vi "Set all current limits (SubVI).vi"() -> (3 "String":string)   [LabVIEW 2018]
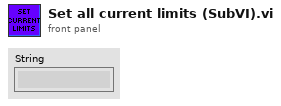
[diagram p1: front panel]
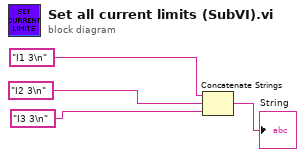
[diagram p0: block diagram]
diagram:
  n1 = Concatenate Strings("I1 3\n", "I2 3\n", "I3 3\n") -> (→"String":string)
